vi "Configuration Files.vi"(8 "error in":errorcluster, 11 "Node Ptr":T1 format="%.0x") -> (0 "error out":errorcluster)   [LabVIEW 2020, in "AIM MIL-STD-1553 System Explorer.lvlib" / "Implementation.lvlib"]
uses:
  Implementation.lvlib
  <vilib>/NI VeriStand/Custom Device API/Custom Device Item Ref.ctl
  <vilib>/NI VeriStand/Custom Device API/Custom Device API.lvlib
  Scripting/AIM MIL-STD-1553 Scripting.lvlib
  Refresh/Refresh.lvlib
panel:
  in  "Create Tx/Rx Folders for Subaddresses?":bool
  in  "refresh":bool
  in  "parameter config file path":path caption="Parameter Configuration File Path"
  in  "SHDocVw.IWebBrowser":refnum<k7>(container)
  in  "General Header":cluster{"Section Name":string}={"Section Name"="MIL-STD-1553 - Configuration Files"}
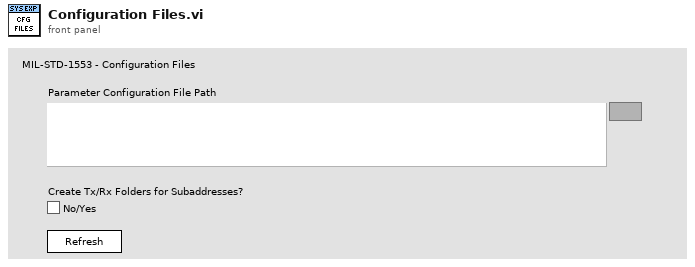
[diagram p1: front panel]
types:
  T1 = typedef "Custom Device API.lvlib/Custom Device Item Ref.ctl" = u64
  T2 = typedef "Custom Device API.lvlib/Custom Device Commands.ctl" = enum16{"Default", "Item renamed", "Shutdown", "Dynamic button pressed"}
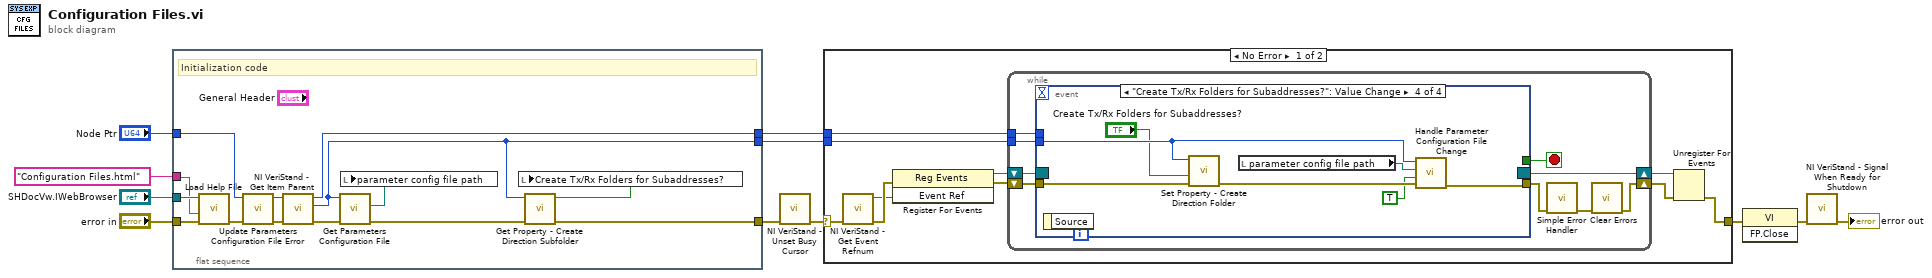
[diagram p0: block diagram]
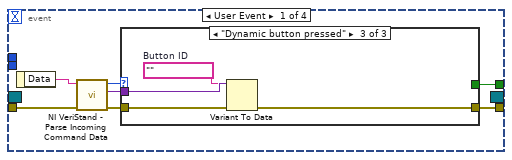
[diagram p2: hidden frame]
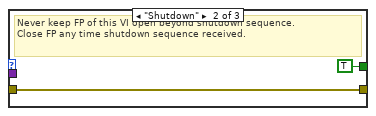
[diagram p4: hidden frame]
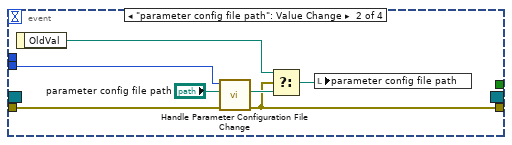
[diagram p5: hidden frame]
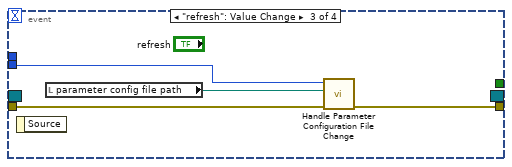
[diagram p6: hidden frame]
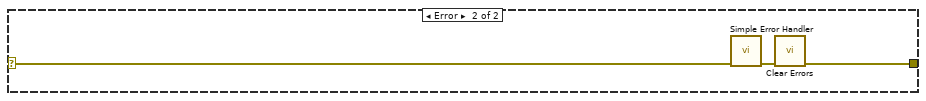
[diagram p7: hidden frame]
diagram:
  n1 = flat-sequence "Initialization code" {
    tunnel: "error in" -> [w25]
    tunnel: "Node Ptr" -> [w20]
    tunnel: [w15] -> w7
    tunnel: "SHDocVw.IWebBrowser" -> [w24]
    tunnel: "Configuration Files.html" ("CD_CHM_Section") -> [w13]
    tunnel: [w14] -> w2
    tunnel: [w21] -> w1
    frame #0 {
      # "Initialization code"
      n2 = call "Load Help File.vi"("error in (no error)"=w25, "HTML File to Load"=w13, "Browser"=w24) -> ("error out"=w17:errorcluster)  [unwired: 8 in]
      n3 = call "Update Parameters Configuration File Error.vi"("error in"=w17, "configuration files section"=w20) -> ("error out"=w19:errorcluster, "configuration files section out"=w18:T1)  [unwired: 8 in]
      n4 = call <vilib>:"NI VeriStand - Get Item Parent.vi"("error in (no error)"=w19, "Item Ref in"=w18) -> ("error out"=w23:errorcluster, "Parent Ref"=w14:T1, "Item Ref out"=w21:T1)  [unwired: 6 in, 1 out]
      n5 = call "Get Parameters Configuration File.vi"("error in"=w23, "custom device"=w14) -> ("error out"=w16:errorcluster, "parameters configuration file"=w22:path)  [unwired: 6 in, 2 out]
      n6 = local write "parameter config file path"(w22) -> ()
      n7 = call "Get Property - Create Direction Subfolder.vi"("error in"=w16, "custom device"=w14) -> ("error out"=w15:errorcluster, "Value"=w12:bool)  [unwired: 8 in]
      n8 = local write "Create Tx/Rx Folders for Subaddresses?"(w12) -> ()
    }
  }
  n9 = call <vilib>:"NI VeriStand - Unset Busy Cursor.vi"("error in (no error)"=w7) -> ("error out"=w6:errorcluster)  [unwired: 10 out]
  n10 = case shown="No Error" w6 {
    selector: w6 -> [w28 w79]
    tunnel: [w32 w77] -> w11
    tunnel: w2 -> [w27 _]
    tunnel: w1 -> [w26 _]
    frame No Error {
      n11 = call <vilib>:"NI VeriStand - Get Event Refnum.vi"("error in (no error)"=w28) -> ("error out"=w35:errorcluster, "Event Ref"=w31:refnum<user-event>)  [unwired: 9 out]
      n12 = register-events(error in=w35, w31) -> (reference out=w29:refnum<event-registration>, error out=w30:errorcluster)  [unwired: 1 in]
      n13 = while {
        shift-right: [w38] -> w33
        shift-left: w30 -> [w43]
        shift-right: [w44] -> w34
        shift-left: w29 -> [w42]
        tunnel: w27 -> [w37]
        tunnel: w26 -> [w36]
        stop <- w41 stop-if-true
        n14 = event shown="[3] \"Create Tx/Rx Folders for Subaddresses?\": Value Change" {
          selector: w42 -> [_ _ _ _]
          dyn-events: [_ _ _ _] -> w44
          timeout: _ -> [_ _ _ _]
          tunnel: w43 -> [w51 w65 w68 w76]
          tunnel: [w48 _ _ _] -> w41
          tunnel: [w47 w61 w69 w74] -> w40
          tunnel: w37 -> [_ w64 w67 w73]
          tunnel: w36 -> [_ _ _ _]
          event User Event {
            n15 = event-data() -> ("Data"=w45:string)  [unwired: 1 out]
            n16 = call <vilib>:"NI VeriStand - Parse Incoming Command Data.vi"("error in (no error)"=w51, "Incoming data"=w45) -> ("error out"=w50:errorcluster, "Outgoing data"=w46:variant, "Action"=w49:T2)  [unwired: 7 out]
            n17 = case shown="\"Dynamic button pressed\"" w49 {
              tunnel: w50 -> [w52 w53 w58]
              tunnel: [_ TRUE _] -> w48
              tunnel: [w52 w53 w55] -> w47
              tunnel: w46 -> [_ _ w57]
              frame Default {
                # "Ignore"
              }
              frame "Shutdown" {
                # "Never keep FP of this VI open beyond shutdown sequence.\nClose FP any time shutdown sequence received."
              }
              frame "Dynamic button pressed" {
                w56 = ""  # Button ID
                n18 = Variant To Data(error in=w58, type=w56, Variant=w57) -> (error out=w55:errorcluster)  [unwired: 1 out]
              }
            }
          }
          event "parameter config file path": Value Change {
            n19 = event-data() -> ("OldVal"=w60:path)  [unwired: 1 out]
            n20 = call "Handle Parameter Configuration File Change.vi"("error in"=w65, "new parameter configuration file path"="parameter config file path", "custom device ref"=w64) -> ("error out"=w61:errorcluster, "parameters configuration file out"=w62:path)  [unwired: 6 in, 1 out]
            n21 = Select(t=w60, s=w61, f=w62) -> (s? t:f=w59:path)
            n22 = local write "parameter config file path"(w59) -> ()
          }
          event "refresh": Value Change {
            n23 = event-data() -> ()  [unwired: 2 out]
            n24 = local read "parameter config file path"() -> (w66:path)
            n25 = call "Handle Parameter Configuration File Change.vi"("error in"=w68, "new parameter configuration file path"=w66, "custom device ref"=w67) -> ("error out"=w69:errorcluster)  [unwired: 6 in, 2 out]
          }
          event "Create Tx/Rx Folders for Subaddresses?": Value Change {
            n26 = event-data() -> ()  [unwired: 2 out]
            n27 = call "Set Property - Create Direction Folder.vi"("error in"=w76, "create Tx/Rx folders for subaddresses?"="Create Tx/Rx Folders for Subaddresses?", "custom device"=w73) -> ("error out"=w75:errorcluster)  [unwired: 7 in, 1 out]
            n28 = local read "parameter config file path"() -> (w72:path)
            n29 = call "Handle Parameter Configuration File Change.vi"("error in"=w75, "create Tx/Rx folders for subaddresses value change?"=TRUE ("include direction section"), "new parameter configuration file path"=w72, "custom device ref"=w73) -> ("error out"=w74:errorcluster)  [unwired: 5 in, 2 out]
          }
        }
        n30 = call <vilib>:"Simple Error Handler.vi"("error in (no error)"=w40) -> ("error out"=w39:errorcluster)  [unwired: 1 in, 7 out]
        n31 = call <vilib>:"Clear Errors.vi"("error in (no error)"=w39) -> ("error out"=w38:errorcluster)  [unwired: 1 in, 5 out]
      }
      n32 = Unregister For Events(event registration refnum=w34, error in=w33) -> (error out=w32:errorcluster)
    }
    frame Error {
      n33 = call <vilib>:"Simple Error Handler.vi"("error in (no error)"=w79) -> ("error out"=w78:errorcluster)  [unwired: 1 in, 7 out]
      n34 = call <vilib>:"Clear Errors.vi"("error in (no error)"=w78) -> ("error out"=w77:errorcluster)  [unwired: 1 in, 5 out]
    }
  }
  n35 = invoke class="VI" method="FP.Close"(error in=w11) -> (error out=w10:errorcluster)  [unwired: 2 in, 2 out]
  n36 = call <vilib>:"NI VeriStand - Signal When Ready for Shutdown.vi"("error in (no error)"=w10) -> ("error out"=→"error out":errorcluster)  [unwired: 10 out]
